vi "Write DefaultPythonVersion.vi"(8 "error in (no error)":errorcluster, 10 "DefaultPythonVersion":string="3.9", 11 "ArgparseWrapper in":refnum<class "ArgparseWrapper.lvclass">) -> (0 "error out":errorcluster, 3 "ArgparseWrapper out":refnum<class "ArgparseWrapper.lvclass">)   [LabVIEW 2022 SP3, in "ArgumentParser.lvlib" / "ArgparseWrapper.lvclass"]
uses:
  ArgparseWrapper.lvclass
  ArgparseWrapper.lvclass/ArgparseWrapper.ctl
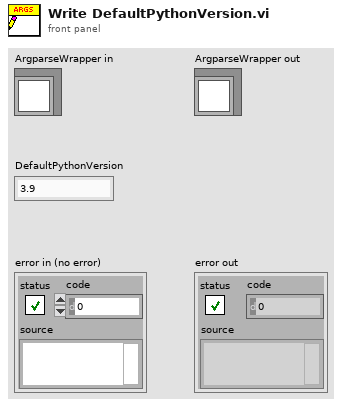
[diagram p1: front panel]
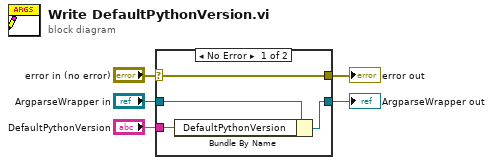
[diagram p0: block diagram]
diagram:
  n1 = case shown="No Error" "error in (no error)" {
    selector: "error in (no error)" -> [w9 w10]
    tunnel: [w9 w10] -> w4
    tunnel: [w7 w11] -> w2
    tunnel: "ArgparseWrapper in" -> [w8 w11]
    tunnel: "DefaultPythonVersion" -> [w6 _]
    frame No Error {
      n2 = Bundle By Name(cluster=w8, "DefaultPythonVersion"=w6) -> (w7:refnum<class "ArgparseWrapper.lvclass">)
    }
    frame Error {
    }
  }
  "error out" <- w4
  "ArgparseWrapper out" <- w2
